vi "CosmeticCleanup.vi"(8 "error in (no error)":errorcluster, 11 "BaseAccessorScripter in":refnum<class "BaseAccessorScripter.lvclass">) -> (0 "error out":errorcluster, 3 "BaseAccessorScripter out":refnum<class "BaseAccessorScripter.lvclass">)   [LabVIEW 2021, in "MemberVICreation.lvlib" / "BaseAccessorScripter.lvclass"]
uses:
  <resource>/Framework/Providers/LVClassLibrary/NewAccessors/BaseAccessorScripter/BaseAccessorScripter.lvclass
  <resource>/Framework/Providers/LVClassLibrary/NewAccessors/BaseAccessorScripter/BaseAccessorScripter.lvclass/BaseAccessorScripter.ctl
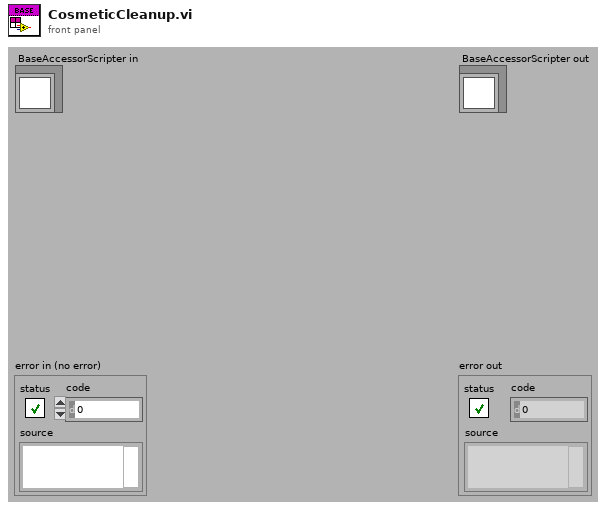
[diagram p1: front panel]
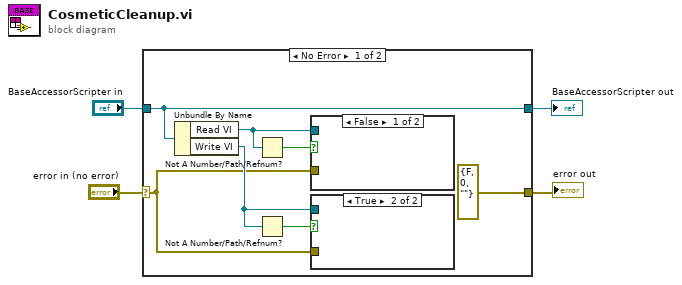
[diagram p0: block diagram]
diagram:
  n1 = case shown="No Error" "error in (no error)" {
    selector: "error in (no error)" -> [w6 w13]
    tunnel: [errorcluster {"status"=FALSE, "code"=0, "source"=""} ("error out") w13] -> w3
    tunnel: [w11 w12] -> w1
    tunnel: "BaseAccessorScripter in" -> [w11 w12]
    frame No Error {
      n2 = Unbundle By Name(w11) -> ("Read VI"=w8:refnum<vi>, "Write VI"=w7:refnum<vi>)
      n3 = Not A Number/Path/Refnum?(number/path/refnum=w8) -> (NaN/Path/Refnum?=w10:bool)
      n4 = Not A Number/Path/Refnum?(number/path/refnum=w7) -> (NaN/Path/Refnum?=w9:bool)
      n5 = case shown="False" w10 {
        tunnel: w8 -> [_ _]
        tunnel: w6 -> [_ _]
        frame False {
        }
        frame True {
        }
      }
      n6 = case shown="True" w9 {
        tunnel: w7 -> [_ _]
        tunnel: w6 -> [_ _]
        frame False {
        }
        frame True {
        }
      }
    }
    frame Error {
    }
  }
  "error out" <- w3
  "BaseAccessorScripter out" <- w1
